vi "DiffDrivePoseEst2_AddVisionMeasurement.vi"(9 "TImeStamp_Seconds":dbl=0.02, 10 "visionRobotPose":T6={"TRANSLATION"={"X"=0.0, "Y"=0.0}, "ROTATION"={"VALUE"=0.0, "COS"=1.0, "SIN"=0.0}} {"ROTATION"."SIN" format="%13.4f"; "ROTATION"."COS" format="%13.4f"; "ROTATION"."VALUE" format="%13.4f"; "TRANSLATION"."Y" format="%14.3f"; "TRANSLATION"."X" format="%14.3f"}, 11 "in DiffDrivePoseEst2":T1={"M_Vision_K"=[], "m_nominal_dT"=0.0, "m_PrevTime_Sec"=0.0, "Pose_Buffer"={"TimeStamps"=[], "DataArray"=[], "Min_TimeStamp"=0.0, "Max_TimeStamp"=0.0, "ItemCount"=0, "MaxBufferTime"=0.0}, "Diff_Drive_Kinematics"={"TrackWidth_Meters"=0.0}, "Diff_Drive_Odom_2"={"M_POSE_Meters"={"TRANSLATION"={"X"=0.0, "Y"=0.0}, "ROTATION"={"VALUE"=0.0, "COS"=1.0, "SIN"=0.0}}, "M_GyroOffset"={"VALUE"=0.0, "COS"=1.0, "SIN"=0.0}, "M_PrevAngle"={"VALUE"=0.0, "COS"=1.0, "SIN"=0.0}, "M_PrevLeftDist_M"=0.0, "M_PrevRightDist_M"=0.0, "M_InitLeftDist_M"=0.0, "M_InitRightDist_M"=0.0}, "M_Q"=[[0.0], [0.0], [0.0]]} {"Diff_Drive_Odom_2"."M_PrevAngle"."SIN" format="%13.4f"; "Diff_Drive_Odom_2"."M_PrevAngle"."COS" format="%13.4f"; "Diff_Drive_Odom_2"."M_PrevAngle"."VALUE" format="%13.4f"; "Diff_Drive_Odom_2"."M_GyroOffset"."SIN" format="%13.4f"; "Diff_Drive_Odom_2"."M_GyroOffset"."COS" format="%13.4f"; "Diff_Drive_Odom_2"."M_GyroOffset"."VALUE" format="%13.4f"; "Diff_Drive_Odom_2"."M_POSE_Meters"."ROTATION"."SIN" format="%13.4f"; "Diff_Drive_Odom_2"."M_POSE_Meters"."ROTATION"."COS" format="%13.4f"; "Diff_Drive_Odom_2"."M_POSE_Meters"."ROTATION"."VALUE" format="%13.4f"; "Diff_Drive_Odom_2"."M_POSE_Meters"."TRANSLATION"."Y" format="%14.3f"; "Diff_Drive_Odom_2"."M_POSE_Meters"."TRANSLATION"."X" format="%14.3f"; "Diff_Drive_Kinematics"."TrackWidth_Meters" format="%20.4f"}) -> (0 "Error":bool, 3 "Out DiffDrivePoseEst2":T1={"M_Vision_K"=[], "m_nominal_dT"=0.0, "m_PrevTime_Sec"=0.0, "Pose_Buffer"={"TimeStamps"=[], "DataArray"=[], "Min_TimeStamp"=0.0, "Max_TimeStamp"=0.0, "ItemCount"=0, "MaxBufferTime"=0.0}, "Diff_Drive_Kinematics"={"TrackWidth_Meters"=0.0}, "Diff_Drive_Odom_2"={"M_POSE_Meters"={"TRANSLATION"={"X"=0.0, "Y"=0.0}, "ROTATION"={"VALUE"=0.0, "COS"=1.0, "SIN"=0.0}}, "M_GyroOffset"={"VALUE"=0.0, "COS"=1.0, "SIN"=0.0}, "M_PrevAngle"={"VALUE"=0.0, "COS"=1.0, "SIN"=0.0}, "M_PrevLeftDist_M"=0.0, "M_PrevRightDist_M"=0.0, "M_InitLeftDist_M"=0.0, "M_InitRightDist_M"=0.0}, "M_Q"=[[0.0], [0.0], [0.0]]} {"Diff_Drive_Odom_2"."M_PrevAngle"."SIN" format="%13.4f"; "Diff_Drive_Odom_2"."M_PrevAngle"."COS" format="%13.4f"; "Diff_Drive_Odom_2"."M_PrevAngle"."VALUE" format="%13.4f"; "Diff_Drive_Odom_2"."M_GyroOffset"."SIN" format="%13.4f"; "Diff_Drive_Odom_2"."M_GyroOffset"."COS" format="%13.4f"; "Diff_Drive_Odom_2"."M_GyroOffset"."VALUE" format="%13.4f"; "Diff_Drive_Odom_2"."M_POSE_Meters"."ROTATION"."SIN" format="%13.4f"; "Diff_Drive_Odom_2"."M_POSE_Meters"."ROTATION"."COS" format="%13.4f"; "Diff_Drive_Odom_2"."M_POSE_Meters"."ROTATION"."VALUE" format="%13.4f"; "Diff_Drive_Odom_2"."M_POSE_Meters"."TRANSLATION"."Y" format="%14.3f"; "Diff_Drive_Odom_2"."M_POSE_Meters"."TRANSLATION"."X" format="%14.3f"; "Diff_Drive_Kinematics"."TrackWidth_Meters" format="%20.4f"})   [LabVIEW 2019, in "Trajectory_Library.lvlib"]
doc: "Add a vision measurement to the Unscented Kalman Filter. This will correct the odometry pose estimate while still accounting for measurement noise.\n \nThis method can be called as infrequently as you want, as long as you are calling DifferentialDrivePoseEstimator_update every loop.\n\nTo promote stability of the pose estimate and make it robust to bad vision data, we recommend only adding vision measurements that are already within one meter or so of the current pose estimate.\n\n Inputs:\n - InDIffDrivePoseEstimate -- Data cluster for this system\n - visionRobotPoseMeters -- The pose of the robot as measured by the vision camera.\n - timestampSeconds -- The timestamp of the vision measurement in seconds. Note that if you don't use your own time source by calling DifferentialDrivePoseEstimator_updateWithTime then you must use a timestamp with an epoch since FPGA startup (i.e. the epoch of this timestamp is the same epoch as Timer.getFPGATimestamp.) This means that you should use Timer.getFPGATimestamp as your time source in this case.\n\nOutputs:\n - OutDIffDrivePoseEstimate -- Data cluster for this system\n - Error -- Returns TRUE if an error occured."
uses:
  <vilib>/Analysis/Matrix/Datatypes/RealMatrix.ctl
  TypeDef/ROTATION2D.ctl
  TypeDef/POSE2D.ctl
  TypeDef/TRANSLATION2D.ctl
  Pose2d_Interpolate.vi
  Pose2d_RelativeTo.vi
  Transform2d_Create_TransRot.vi
  Translation2d_RotateBy.vi
  Translation2d_Plus.vi
  Rotation2d_Plus.vi
  Pose2d_New_TRRO.vi
  VecBuilder_3x1Fill.vi
  Pose2d_getXYAngle.vi
  Twist2d_GetAll.vi
  Twist2d_Create.vi
  Transform2d_Create_PosePose.vi
  Translation2d_Create.vi
  Rotation2d_RotateBy.vi
  Rotation2d_UnaryMinus.vi
  Translation2d_Minus.vi
  Rotation2d_Minus.vi
  Rotation2d_CreateXY.vi
  Rotation2d_CreateAngle.vi
  Util_CalcDist.vi
  <vilib>/gmath/interp.llb/Search Ordered Table.vi
  Pose2d_Log.vi
  Pose2d_Exp.vi
  Trajectory_Library.lvlib
  DiffDrivePoseEst2_InterpRecord_Interp.vi
  <vilib>/Analysis/Matrix/NI_Matrix.lvlib
  TypeDef/TIME_INTERPOLATABLE_VARIANT.ctl
  TypeDef/DIFF_DRIVE_KINEMATICS.ctl
  TypeDef/DIFF_DRIVE_ODOM2.ctl
  TypeDef/DIFF_DRIVE_POSE_EST2.ctl
panel:
  # "NOT A PARAMETER, JUST A DATA TYPE"
  # "<3, 1>"
  # "<3, 3>"
  # "<3, 1>"
  # "<3, 3>"
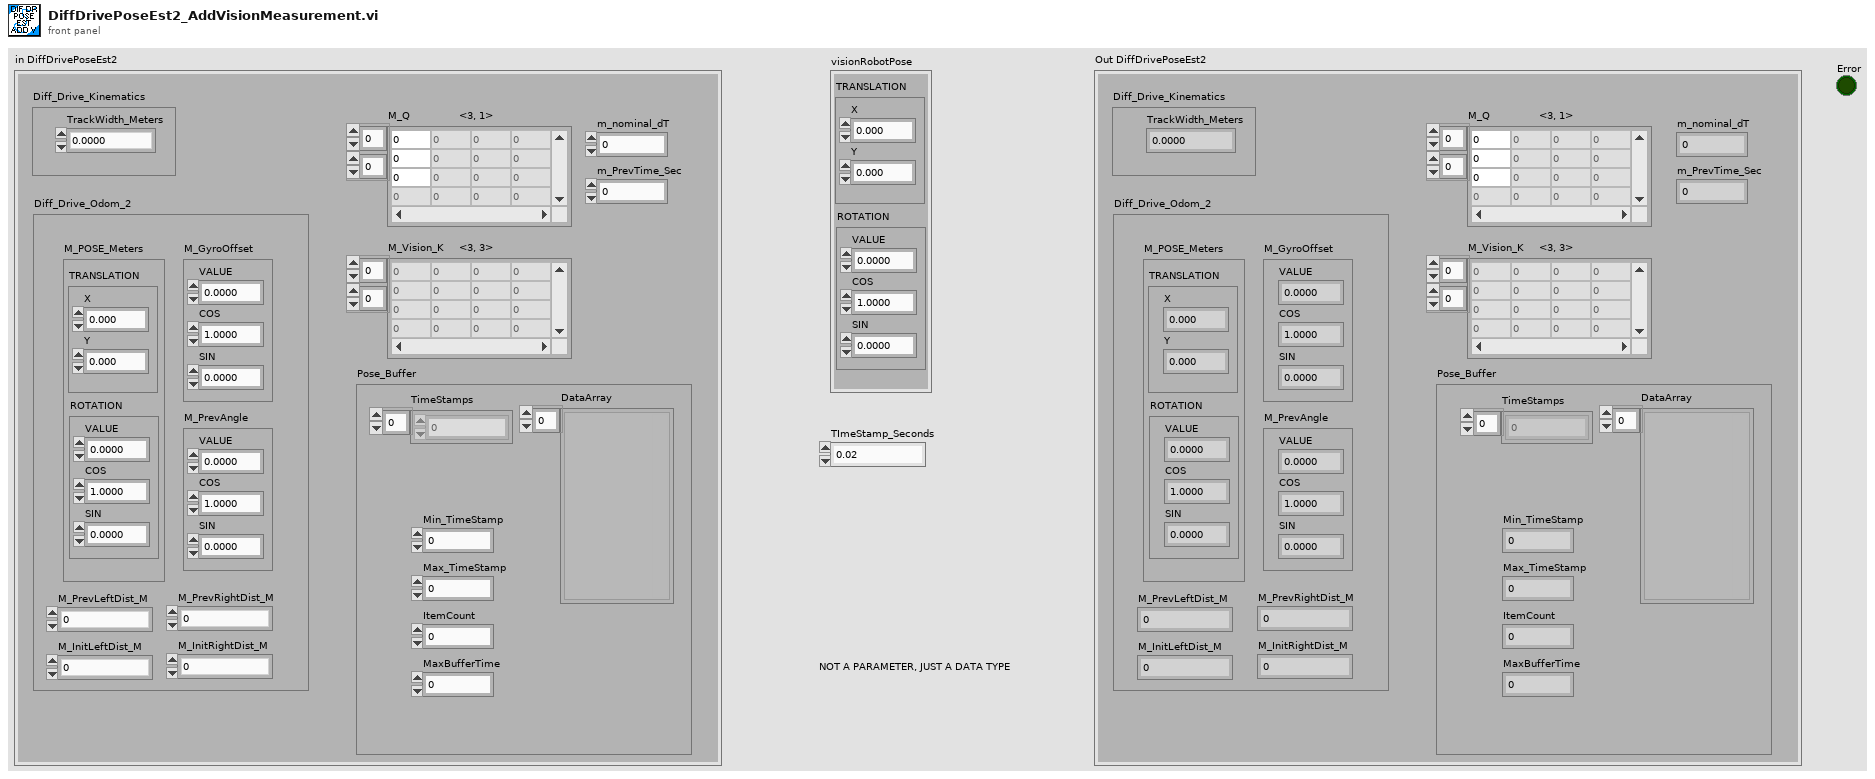
[diagram p1: front panel]
types:
  T1 = typedef "Trajectory_Library.lvlib/DIFF_DRIVE_POSE_EST2.ctl" = cluster{"M_Vision_K":T2, "m_nominal_dT":dbl, "m_PrevTime_Sec":dbl, "Pose_Buffer":T3, "Diff_Drive_Kinematics":T4, "Diff_Drive_Odom_2":T5, "M_Q":T2}
  T2 = typedef "NI_Matrix.lvlib/RealMatrix.ctl" = dbl[][]
  T3 = typedef "Trajectory_Library.lvlib/TIME_INTERPOLATABLE_VARIANT.ctl" = cluster{"TimeStamps":dbl[], "DataArray":variant[], "Min_TimeStamp":dbl, "Max_TimeStamp":dbl, "ItemCount":i32, "MaxBufferTime":dbl}
  T4 = typedef "Trajectory_Library.lvlib/DIFF_DRIVE_KINEMATICS.ctl" = cluster{"TrackWidth_Meters":dbl}
  T5 = typedef "Trajectory_Library.lvlib/DIFF_DRIVE_ODOM2.ctl" = cluster{"M_POSE_Meters":T6, "M_GyroOffset":T8, "M_PrevAngle":T8, "M_PrevLeftDist_M":dbl, "M_PrevRightDist_M":dbl, "M_InitLeftDist_M":dbl, "M_InitRightDist_M":dbl}
  T6 = typedef "Trajectory_Library.lvlib/POSE2D.ctl" = cluster{"TRANSLATION":T7, "ROTATION":T8}
  T7 = typedef "Trajectory_Library.lvlib/TRANSLATION2D.ctl" = cluster{"X":dbl, "Y":dbl}
  T8 = typedef "Trajectory_Library.lvlib/ROTATION2D.ctl" = cluster{"VALUE":dbl, "COS":dbl, "SIN":dbl}
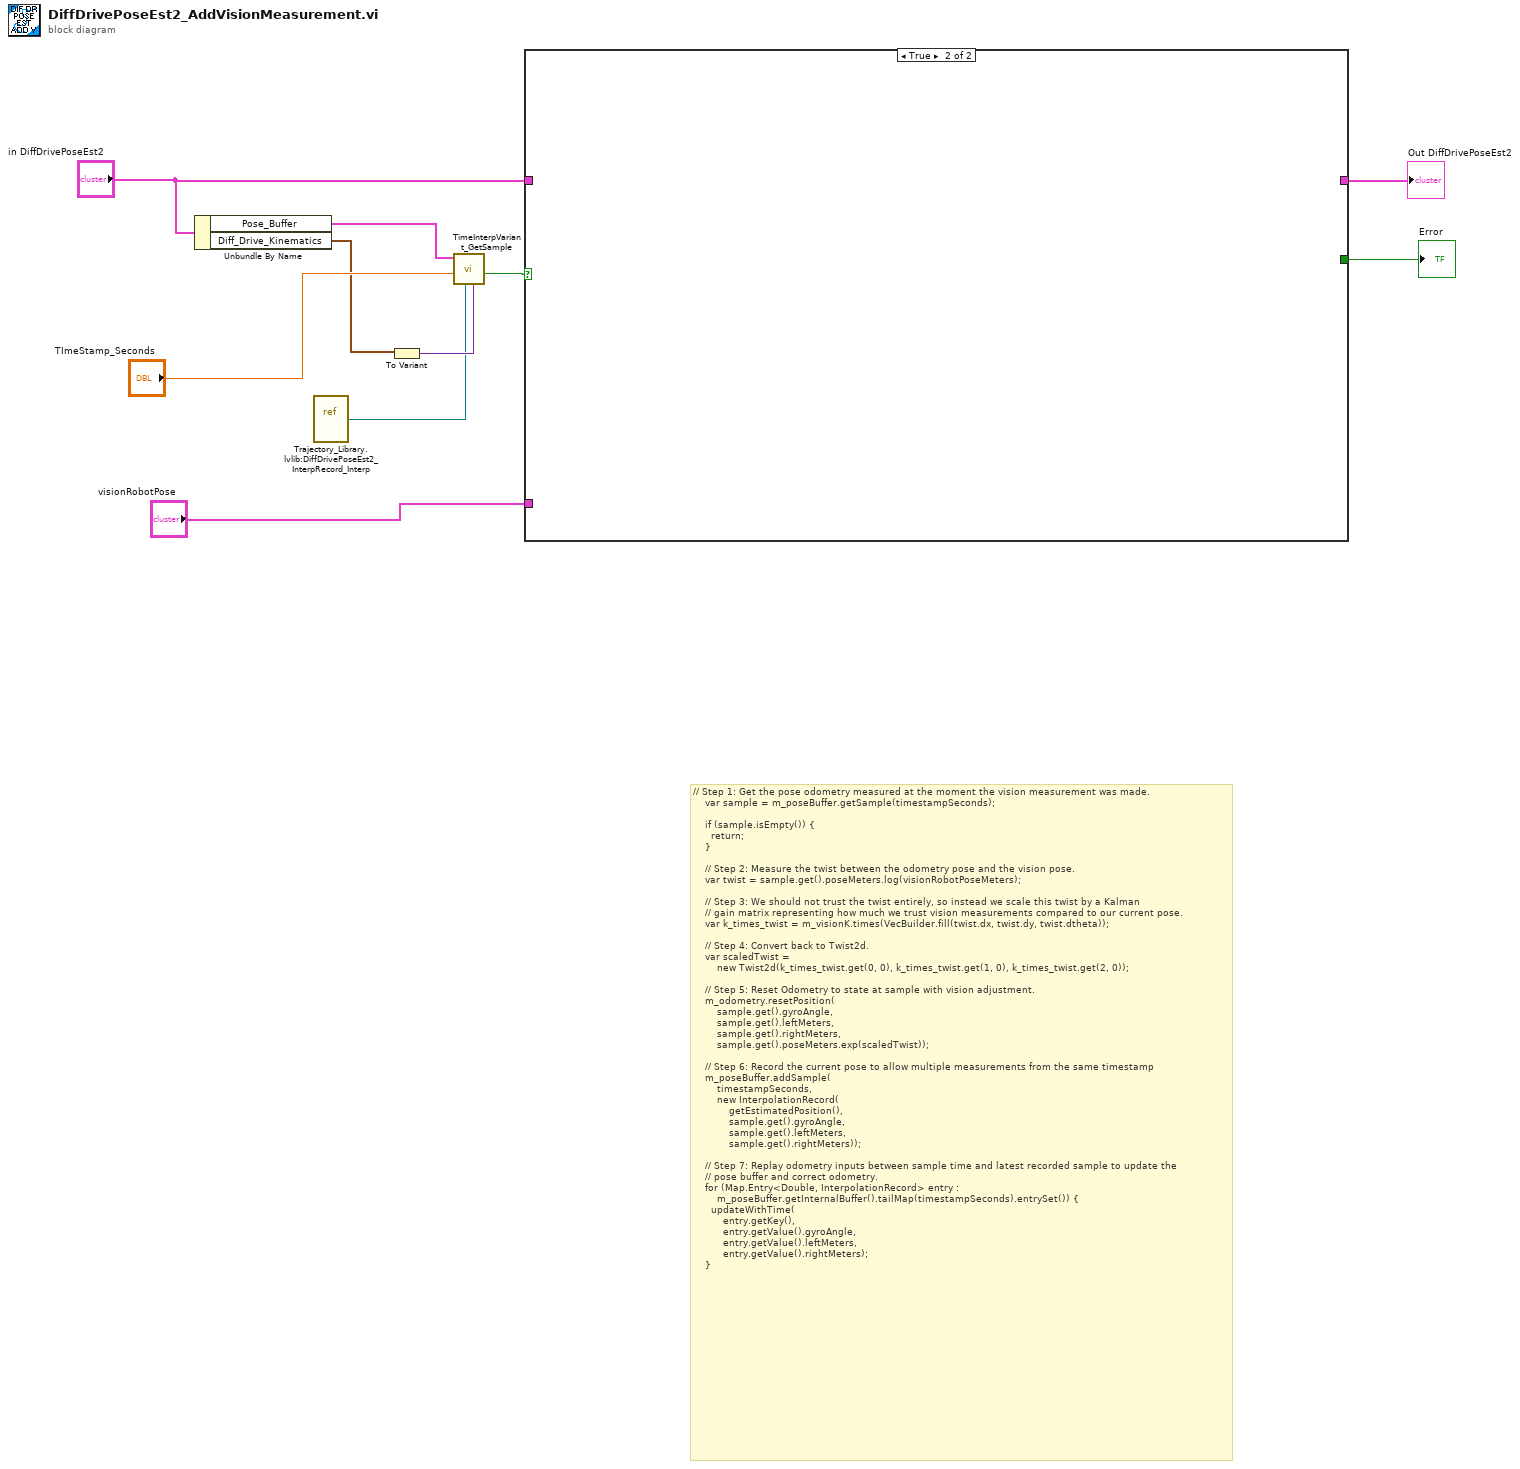
[diagram p0: block diagram]
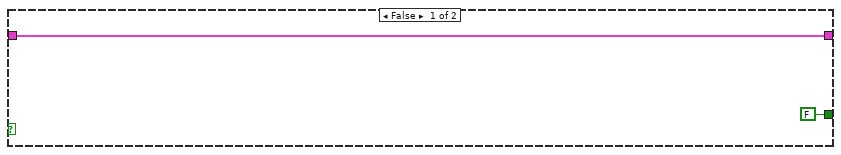
[diagram p2: hidden frame]
diagram:
  # "// Step 1: Get the pose odometry measured at the moment the vision measurement was made.\n    var sample = m_poseBuffer.getSample(timestampSeconds);\n\n    if (sample.isEmpty()) {\n      return;\n    }\n\n    // Step 2: Measure the twist between the odometry pose and the vision pose.\n    var twist = sample.get().poseMeters.log(visionRobotPoseMeters);\n\n    // Step 3: We should not trust the twist entirely, so instead we scale this twist by a Kalman\n    // gain matrix representing how much we trust vision measurements compared to our current pose.\n    var k_times_twist = m_visionK.times(VecBuilder.fill(twist.dx, twist.dy, twist.dtheta));\n\n    // Step 4: Convert back to Twist2d.\n    var scaledTwist =\n        new Twist2d(k_times_twist.get(0, 0), k_times_twist.get(1, 0), k_times_twist.get(2, 0));\n\n    // Step 5: Reset Odometry to state at sample with vision adjustment.\n    m_odometry.resetPosition(\n        sample.get().gyroAngle,\n        sample.get().leftMeters,\n        sample.get().rightMeters,\n        sample.get().poseMeters.exp(scaledTwist));\n\n    // Step 6: Record the current pose to allow multiple measurements from the same timestamp\n    m_poseBuffer.addSample(\n        timestampSeconds,\n        new InterpolationRecord(\n            getEstimatedPosition(),\n            sample.get().gyroAngle,\n            sample.get().leftMeters,\n            sample.get().rightMeters));\n\n    // Step 7: Replay odometry inputs between sample time and latest recorded sample to update the\n    // pose buffer and correct odometry.\n    for (Map.Entry<Double, InterpolationRecord> entry :\n        m_poseBuffer.getInternalBuffer().tailMap(timestampSeconds).entrySet()) {\n      updateWithTime(\n          entry.getKey(),\n          entry.getValue().gyroAngle,\n          entry.getValue().leftMeters,\n          entry.getValue().rightMeters);\n    }"
  n1 = Unbundle By Name("in DiffDrivePoseEst2") -> ("Pose_Buffer"=w6:T3, "Diff_Drive_Kinematics"=w2:T4)
  n2 = vi-ref "Trajectory_Library.lvlib:DiffDrivePoseEst2_InterpRecord_Interp.vi"() -> (w1:refnum<vi>)
  n3 = To Variant(anything=w2) -> (Variant=w3:variant)
  n4 = call "TimeInterpVariant_GetSample.vi"("Extra"=w3, "Interpolate\nReference"=w1, "TimeStamp"="TImeStamp_Seconds", "TimeInterpVariant"=w6) -> ("IsPresent"=w4:bool)  [unwired: 6 in, 1 out]
  n5 = case shown="True" w4 {
    tunnel: [w12 _] -> w10
    tunnel: "visionRobotPose" -> [_ _]
    tunnel: [FALSE _] -> w8
    tunnel: "in DiffDrivePoseEst2" -> [w12 _]
    frame False {
    }
    frame True {
    }
  }
  "Out DiffDrivePoseEst2" <- w10
  "Error" <- w8
